vi "calc_lookup_arrays_from_ideal_spiral.vi"(8 "error in":errorcluster, 9 "Iterations per pixel":u16, 10 "Fiber spiral parameters":T1={"Fiber Frequency"=2200, "Imaging Periods"=100, "Settling Periods"=50, "Resting Periods"=30, "Amplitude X"=0.5, "Amplitude Y"=0.5, "Phase difference"=90.0, "Initial Amplitude X"=0.0, "Initial Amplitude Y"=0.0} {"Initial Amplitude Y" min=0.0 max=3.0 step=0.1; "Initial Amplitude X" min=0.0 max=3.0 step=0.1; "Phase difference" min=0.0 max=360.0 step=5.0; "Amplitude Y" min=0.0 max=3.0 step=0.1; "Amplitude X" min=0.0 max=3.0 step=0.1}, 11 "ImageAssemblerRK110612Spiral in":refnum<class "ImageAssemblerRK110612Spiral.lvclass">) -> (0 "error out":errorcluster, 3 "ImageAssemblerRK110612Spiral out":refnum<class "ImageAssemblerRK110612Spiral.lvclass">)   [LabVIEW 2010, in "ImageAssemblerRK110612Spiral.lvclass"]
uses:
  ImageAssemblerRK110612Spiral.lvclass
  FPGAWrapper/FPGAWrapperRK110512Fiber/FPGAWrapperRK110512Fiber_Spiral/fiber_spiral_parameters.ctl
  ImageAssemblerRK110612Spiral.lvclass/ImageAssemblerRK110612Spiral.ctl
  FPGAWrapper/FPGAWrapperRK110512Fiber/FPGAWrapperRK110512Fiber_Spiral/FPGAWrapperRK110512Fiber_Spiral.lvclass
panel:
  # "[Hz]"
  # "[V]"
  # "[V]"
  # "[deg]"
  # "[V]"
  # "[V]"
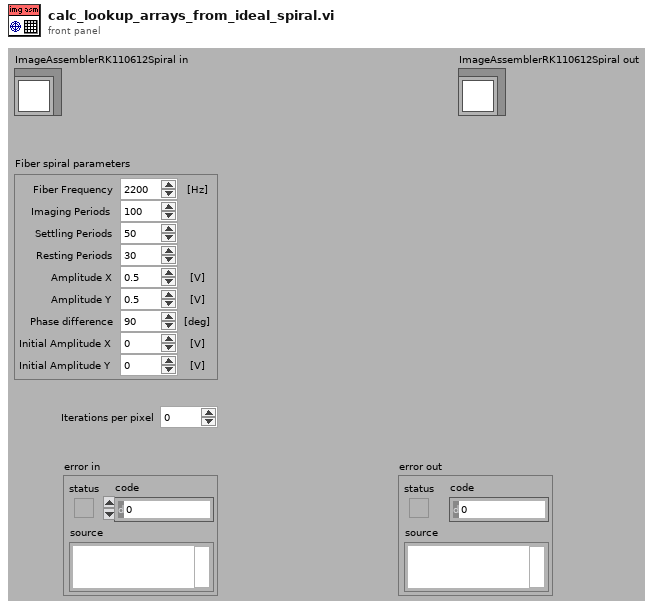
[diagram p1: front panel]
types:
  T1 = typedef "FPGAWrapperRK110512Fiber_Spiral.lvclass/fiber_spiral_parameters.ctl" = cluster{"Fiber Frequency":u16, "Imaging Periods":u16, "Settling Periods":u16, "Resting Periods":u16, "Amplitude X":dbl, "Amplitude Y":dbl, "Phase difference":dbl, "Initial Amplitude X":dbl, "Initial Amplitude Y":dbl}
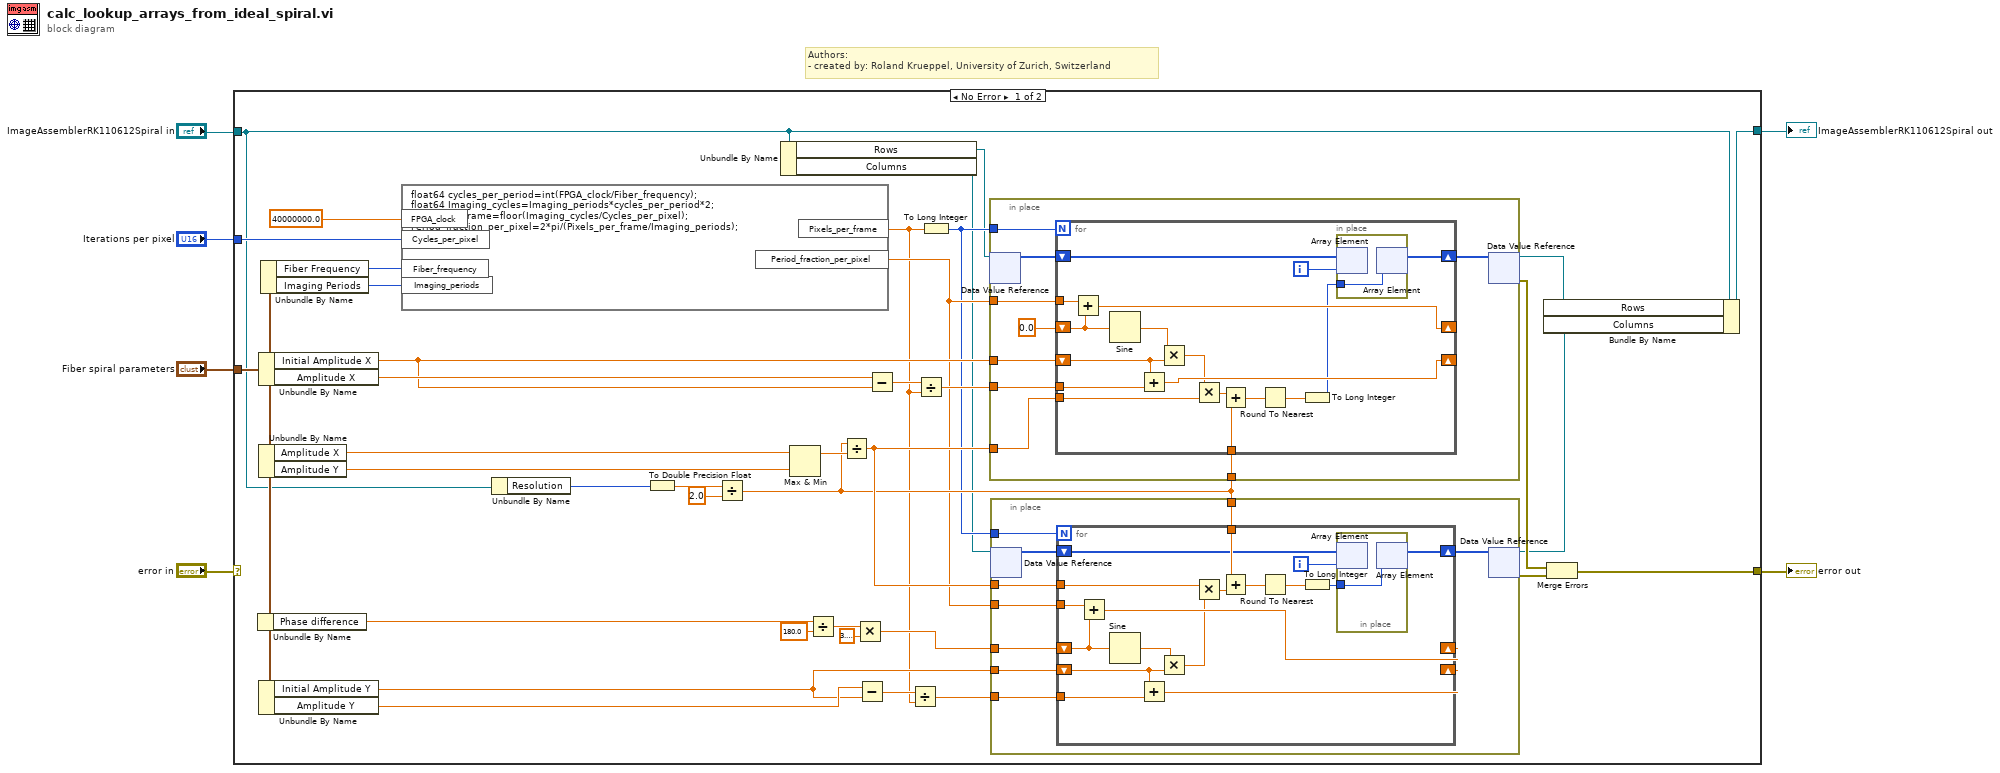
[diagram p0: block diagram]
diagram:
  # "Authors: \n- created by: Roland Krueppel, University of Zurich, Switzerland"
  n1 = case shown="No Error" "error in" {
    selector: "error in" -> [_ w100]
    tunnel: "Fiber spiral parameters" -> [w25 _]
    tunnel: "Iterations per pixel" -> [w24 _]
    tunnel: [w19 w100] -> w4
    tunnel: "ImageAssemblerRK110612Spiral in" -> [w14 w99]
    tunnel: [w13 w99] -> w1
    frame No Error {
      n2 = Unbundle By Name(w25) -> ("Phase difference"=w36:dbl)
      n3 = Unbundle By Name(w25) -> ("Initial Amplitude X"=w43:dbl, "Amplitude X"=w44:dbl)
      n4 = Unbundle By Name(w25) -> ("Amplitude X"=w31:dbl, "Amplitude Y"=w30:dbl)
      n5 = Unbundle By Name(w25) -> ("Initial Amplitude Y"=w37:dbl, "Amplitude Y"=w38:dbl)
      n6 = Unbundle By Name(w25) -> ("Fiber Frequency"=w21:u16, "Imaging Periods"=w22:u16)
      n7 = formula code="float64 cycles_per_period=int(FPGA_clock/Fiber_frequency);\nfloat64 Imaging_cycles=Imaging_periods*cycles_per_period*2;\nPixels_per_frame=floor(Imaging_cycles/Cycles_per_pixel);\nPeriod_fraction_per_pixel=2*pi/(Pixels_per_frame/Imaging_periods);"("Cycles_per_pixel"=w24, "Imaging_periods"=w22, "Fiber_frequency"=w21, "FPGA_clock"=40000000.0 ("input variable")) -> ("Pixels_per_frame"=w16:dbl, "Period_fraction_per_pixel"=w20:dbl)
      n8 = Unbundle By Name(w14) -> ("Resolution"=w15:u16)
      n9 = To Double Precision Float(number=w15) -> (double precision float=w18:dbl)
      n10 = Divide(x=w18, y=2.0) -> (x/y=w26:dbl)
      n11 = Unbundle By Name(w14) -> ("Rows"=w12:refnum<data-value>, "Columns"=w9:refnum<data-value>)
      n12 = Max & Min(x=w31, y=w30) -> (max(x,y)=w29:dbl)  [unwired: 1 out]
      n13 = Divide(x=w36, y=180.0) -> (x/y=w34:dbl)
      n14 = Divide(x=w26, y=w29) -> (x/y=w27:dbl)
      n15 = Multiply(x=w34, y=3.141592653589793) -> (x*y=w32:dbl)
      n16 = Subtract(x=w38, y=w37) -> (x-y=w40:dbl)
      n17 = Subtract(x=w44, y=w43) -> (x-y=w42:dbl)
      n18 = Divide(x=w40, y=w16) -> (x/y=w39:dbl)
      n19 = Divide(x=w42, y=w16) -> (x/y=w41:dbl)
      n20 = To Long Integer(number=w16) -> (32bit integer=w17:i32)
      n21 = in-place {
        in-place-border: w43 -> [w80]
        in-place-border: w41 -> [w79]
        in-place-border: w27 -> [w78]
        in-place-border: w26 -> [w77]
        in-place-border: w20 -> [w76]
        in-place-border: w17 -> [w75]
        n22 = in-place-dvr #1(w12) -> (w74:i32[])  [unwired: 1 out]
        n23 = for {
          N: w75 -> [_]
          shift-right: [w96] -> _
          shift-left: 0.0 ("x") -> [w97]
          tunnel: w76 -> [w95]
          shift-right: [w93] -> _
          shift-left: w80 -> [w92]
          tunnel: w79 -> [w91]
          tunnel: w78 -> [w89]
          tunnel: w77 -> [w88]
          shift-right: [w81] -> w72
          shift-left: w74 -> [w84]
          i -> [w83]
          n24 = Add(x=w95, y=w97) -> (x+y=w96:dbl)
          n25 = Sine(x=w97) -> (sin(x)=w94:dbl)
          n26 = Add(x=w92, y=w91) -> (x+y=w93:dbl)
          n27 = Multiply(x=w94, y=w92) -> (x*y=w90:dbl)
          n28 = Multiply(x=w90, y=w89) -> (x*y=w87:dbl)
          n29 = Add(x=w87, y=w88) -> (x+y=w85:dbl)
          n30 = Round To Nearest(number=w85) -> (nearest integer value=w86:dbl)
          n31 = To Long Integer(number=w86) -> (32bit integer=w82:i32)
          n32 = in-place {
            in-place-border: w82 -> [w98]
            n33 = in-place-array #2(w84, w83) -> ()  [unwired: 1 out]
            n34 = in-place-array #2(w98) -> (w81:i32[])  [unwired: 1 out]
          }
        }
        n35 = in-place-dvr #1(w72) -> (w11:refnum<data-value>, w10:errorcluster)
      }
      n36 = in-place {
        in-place-border: w39 -> [w53]
        in-place-border: w37 -> [w52]
        in-place-border: w32 -> [w51]
        in-place-border: w27 -> [w50]
        in-place-border: w26 -> [w49]
        in-place-border: w20 -> [w48]
        in-place-border: w17 -> [w47]
        n37 = in-place-dvr #3(w9) -> (w46:i32[])  [unwired: 1 out]
        n38 = for {
          N: w47 -> [_]
          shift-right: [w69] -> _
          shift-left: w51 -> [w70]
          tunnel: w48 -> [w68]
          shift-right: [w66] -> _
          shift-left: w52 -> [w65]
          tunnel: w53 -> [w64]
          tunnel: w50 -> [w63]
          tunnel: w49 -> [w61]
          shift-right: [w54] -> w45
          shift-left: w46 -> [w55]
          i -> [w56]
          n39 = Add(x=w68, y=w70) -> (x+y=w69:dbl)
          n40 = Sine(x=w70) -> (sin(x)=w67:dbl)
          n41 = Add(x=w65, y=w64) -> (x+y=w66:dbl)
          n42 = Multiply(x=w67, y=w65) -> (x*y=w62:dbl)
          n43 = Multiply(x=w63, y=w62) -> (x*y=w60:dbl)
          n44 = Add(x=w61, y=w60) -> (x+y=w58:dbl)
          n45 = Round To Nearest(number=w58) -> (nearest integer value=w59:dbl)
          n46 = To Long Integer(number=w59) -> (32bit integer=w57:i32)
          n47 = in-place {
            in-place-border: w57 -> [w71]
            n48 = in-place-array #4(w55, w56) -> ()  [unwired: 1 out]
            n49 = in-place-array #4(w71) -> (w54:i32[])  [unwired: 1 out]
          }
        }
        n50 = in-place-dvr #3(w45) -> (w8:refnum<data-value>, w7:errorcluster)
      }
      n51 = Bundle By Name(cluster=w14, "Rows"=w11, "Columns"=w8) -> (w13:refnum<class "ImageAssemblerRK110612Spiral.lvclass">)
      n52 = Merge Errors(w10, w7) -> (w19:errorcluster)
    }
    frame Error {
    }
  }
  "error out" <- w4
  "ImageAssemblerRK110612Spiral out" <- w1
